vi "Get Hits.vi"(9 "Hit?":bool, 11 "Power":dbl(slide) scale=0.0..10.0) -> (1 "Load Cell Signal":waveform(dbl)(graph) caption="Sine with Uniform Noise", 2 "Hit? Passed Through":bool, 3 "Hit Value":dbl)   [LabVIEW 2014]
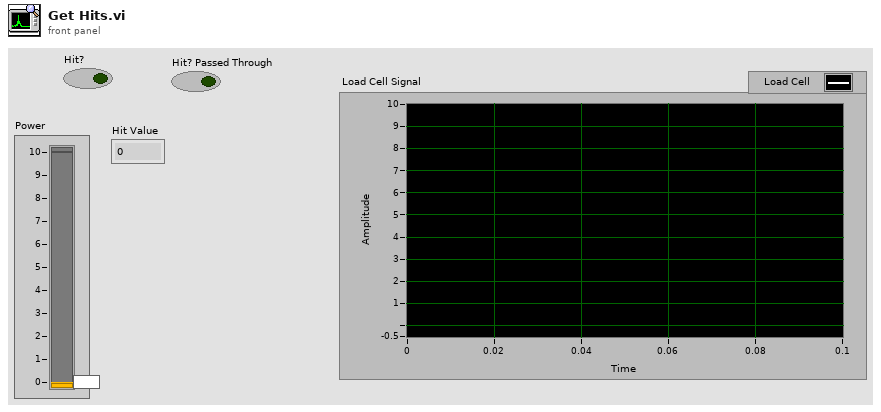
[diagram p1: front panel]
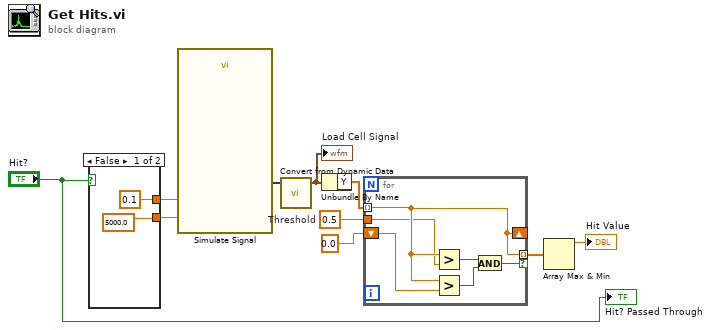
[diagram p0: block diagram]
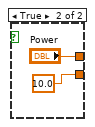
[diagram p2: hidden frame]
diagram:
  w4 = 0.5  # Threshold
  n1 = case shown="False" "Hit?" {
    tunnel: [0.1 ("Vertical Pointer Slide") "Power"] -> w10
    tunnel: [5000.0 ("y") 10.0 ("y")] -> w1
    frame False {
    }
    frame True {
    }
  }
  n2 = call "Simulate Signal"("Frequency"=w1, "Amplitude"=w10) -> ("Load Cell"=w9:dynamicdata)  [unwired: 12 in, 1 out]
  n3 = call "Convert from Dynamic Data"("Dynamic Data Type"=w9) -> ("Waveform"=w6:waveform(dbl))  [unwired: 3 in]
  "Load Cell Signal" <- w6
  n4 = Unbundle By Name(w6) -> ("Y"=w8:dbl[])
  n5 = for {
    shift-right: [w16] -> _
    shift-left: 0.0 ("y") -> [w17]
    tunnel: [w16] -> w5 mode=indexing if=w18
    tunnel: w8 -> [w16] mode=indexing
    tunnel: w4 -> [w15]
    n6 = Greater?(x=w16, y=w15) -> (0:w20:bool)
    n7 = Greater?(x=w16, y=w17) -> (0:w19:bool)
    n8 = And(x=w20, y=w19) -> (x .and. y?=w18:bool)
  }
  n9 = Array Max & Min(array=w5) -> (max value=→"Hit Value":dbl)  [unwired: 3 out]
  "Hit? Passed Through" <- "Hit?"
